vi "002_Control Panel.vi"(11 "Queue Ref In":T1={"UI"=refnum, "Message"=refnum, "Data"=refnum, "Caller"=refnum, "Name"="000 Common", "Data Path"=path "", "Class Path"=path "", "SubPanel"=refnum, "Project Name"="", "MNT"="", "Title"="", "Data Source"=refnum, "Queue List"={}, "VI"=refnum, "UE"=refnum}) -> ()   [LabVIEW 2020]
uses:
  Alin/QMH/000 Module Data Type.ctl
  Alin/QMH/Queue Message.ctl
  <vilib>/Utility/miscctls.llb/LVPointTypeDef.ctl
  0007 Controls/Data Modules.ctl
  0007 Controls/Data Element Single.ctl
  393dfcde-afa0-436b-95a7-8b638b76bd89.vi
  <vilib>/Utility/file.llb/Read Delimited Spreadsheet (string).vi
  <vilib>/Utility/file.llb/Write Delimited Spreadsheet (string).vi
panel:
  in  "Panel Show":bool
  in  "BG3":bool
  in  "BG2":bool
  in  "BG1":bool
  in  "Control Panel":T2
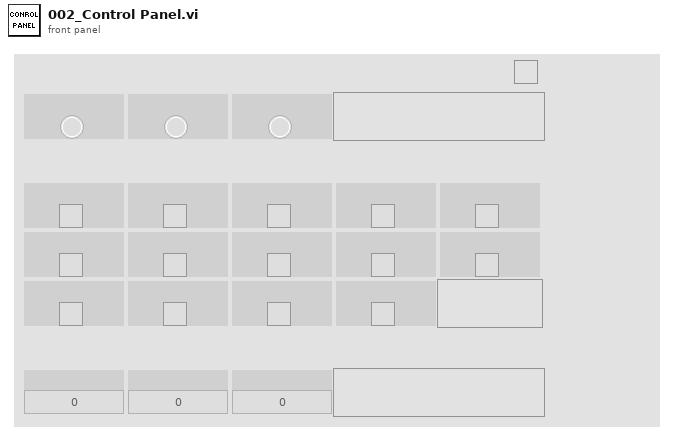
[diagram p1: front panel]
types:
  T1 = typedef "000 Module Data Type.ctl" = cluster{"UI":refnum<queue>, "Message":refnum<queue>, "Data":refnum<queue>, "Caller":refnum<queue>, "Name":string, "Data Path":path, "Class Path":path, "SubPanel":refnum<vi>, "Project Name":string, "MNT":string, "Title":string, "Data Source":refnum<queue>, "Queue List":map{string, refnum<queue>}, "VI":refnum<vi>, "UE":refnum<user-event>}
  T2 = cluster{"System Status":cluster{"Module Name":string, "Data":cluster{"Identifier":string, "Name":string, "Value":bool}[][]}, "Switch":cluster{"Module Name":string, "Data":cluster{"Identifier":string, "Name":string, "Value":bool}[][]}, "Parameter":cluster{"Module Name":string, "Data":cluster{"Identifier":string, "Name":string, "Value":dbl}[][]}}
  T3 = cluster{"Queue":T1, "Array":cluster{string[][]}[], "Active Row":i32, "Delay":cluster{"Count Time(ms)":u32, "Delay Time(ms)":u32, "Next":string}, "Data":cluster{cluster{"Identifier":string, "Name":string, "Value":variant}[][]}[]}
  T4 = typedef "SDQ Data Type.ctl" = cluster{"CAN Length":string, "CAN Name":string, "CAN ID":string, "CAN Type":string, "Test Item":string, "Byte Order":string, "Instruction":string, "Control Type":string, "Group":string, "Offset":dbl, "Coefficient":dbl, "Write Enable":bool, "Lable Type":string, "Key?":string, "Set Value":string, "Upper":dbl, "Lower":dbl, "Unit":string, "Formula":string, "Test Item Type":string, "Length":i32, "Address":string, "Name":string, "Identifier":string, "Data Type":string, "Enumerate?":string, "Enumerate List":string, "Data":string, "Source":string}
  T5 = cluster{cluster{"Identifier":string, "Name":string, "Value":variant}[][]}[]
  T6 = cluster{cluster{"Identifier":string, "Name":string, "Value":variant}[][]}
  T7 = cluster{"Identifier":string, "Name":string, "Value":bool}[][]
  T8 = cluster{"Identifier":string, "Name":string, "Value":dbl}[][]
  T9 = cluster{"Identifier":string, "Name":string, "Value":variant}[][]
  T10 = cluster{"Identifier":string, "Name":string, "Value":bool}
  T11 = cluster{"Identifier":string, "Name":string, "Value":dbl}
  T12 = typedef "eventvkey.ctl" = enum16{"ASCII", "Enter", "Return", "Shift", "Ctrl", "Alt", "Cmd", "Opt", "Caps", "NumLock", "Clear", "Break", "Up", "Down", "Left", "Right", "Insert", "Delete", "Home", "End", "PageUp", "PageDown", "Escape", "Help", "Pause", "ScrollLock", "F1", "F2", "F3", "F4", "F5", "F6", "F7", "F8", "F9", "F10", "F11", "F12", "F13", "F14", "F15", "F16", "F17", "F18", "F19", "F20", "F21", "F22", "F23", "F24", "Play", "VolumeUp", "VolumeDown", "Mute", "Two Byte Char"}
  T13 = cluster{"Shift":bool, "Ctrl":bool, "Alt":bool, "Cmd":bool, "Opt":bool}
  T14 = cluster{"Queue":T1, "Control Panel":refnum<vi>, "Main":refnum<vi>}
  T15 = enum16{"Always On", "Always Off", "Off While Running"}
  T16 = typedef "LVPointTypeDef.ctl" = cluster{"Horizontal":i16, "Vertical":i16}
  T17 = typedef "Data Modules.ctl" = cluster{"Names":cluster{"Module Name":string, "Set Value":string, "Real Value":string, "FB Value":string, "Unit":string, "Identifier":string, "IdentifierW":string, "Decimal":string, "AS":bool, "AR":bool, "Con":bool}, "Data":T18[], "Digit":dbl}
  T18 = typedef "Data Element Single.ctl" = cluster{"Name":string, "Set Value":string, "Real Value":string, "FB Value":string, "Unit":string, "Identifier":string, "Write Name":string, "Decimal":u16, "AS":bool, "AR":bool, "ALM":bool, "Up":bool, "Down":bool}
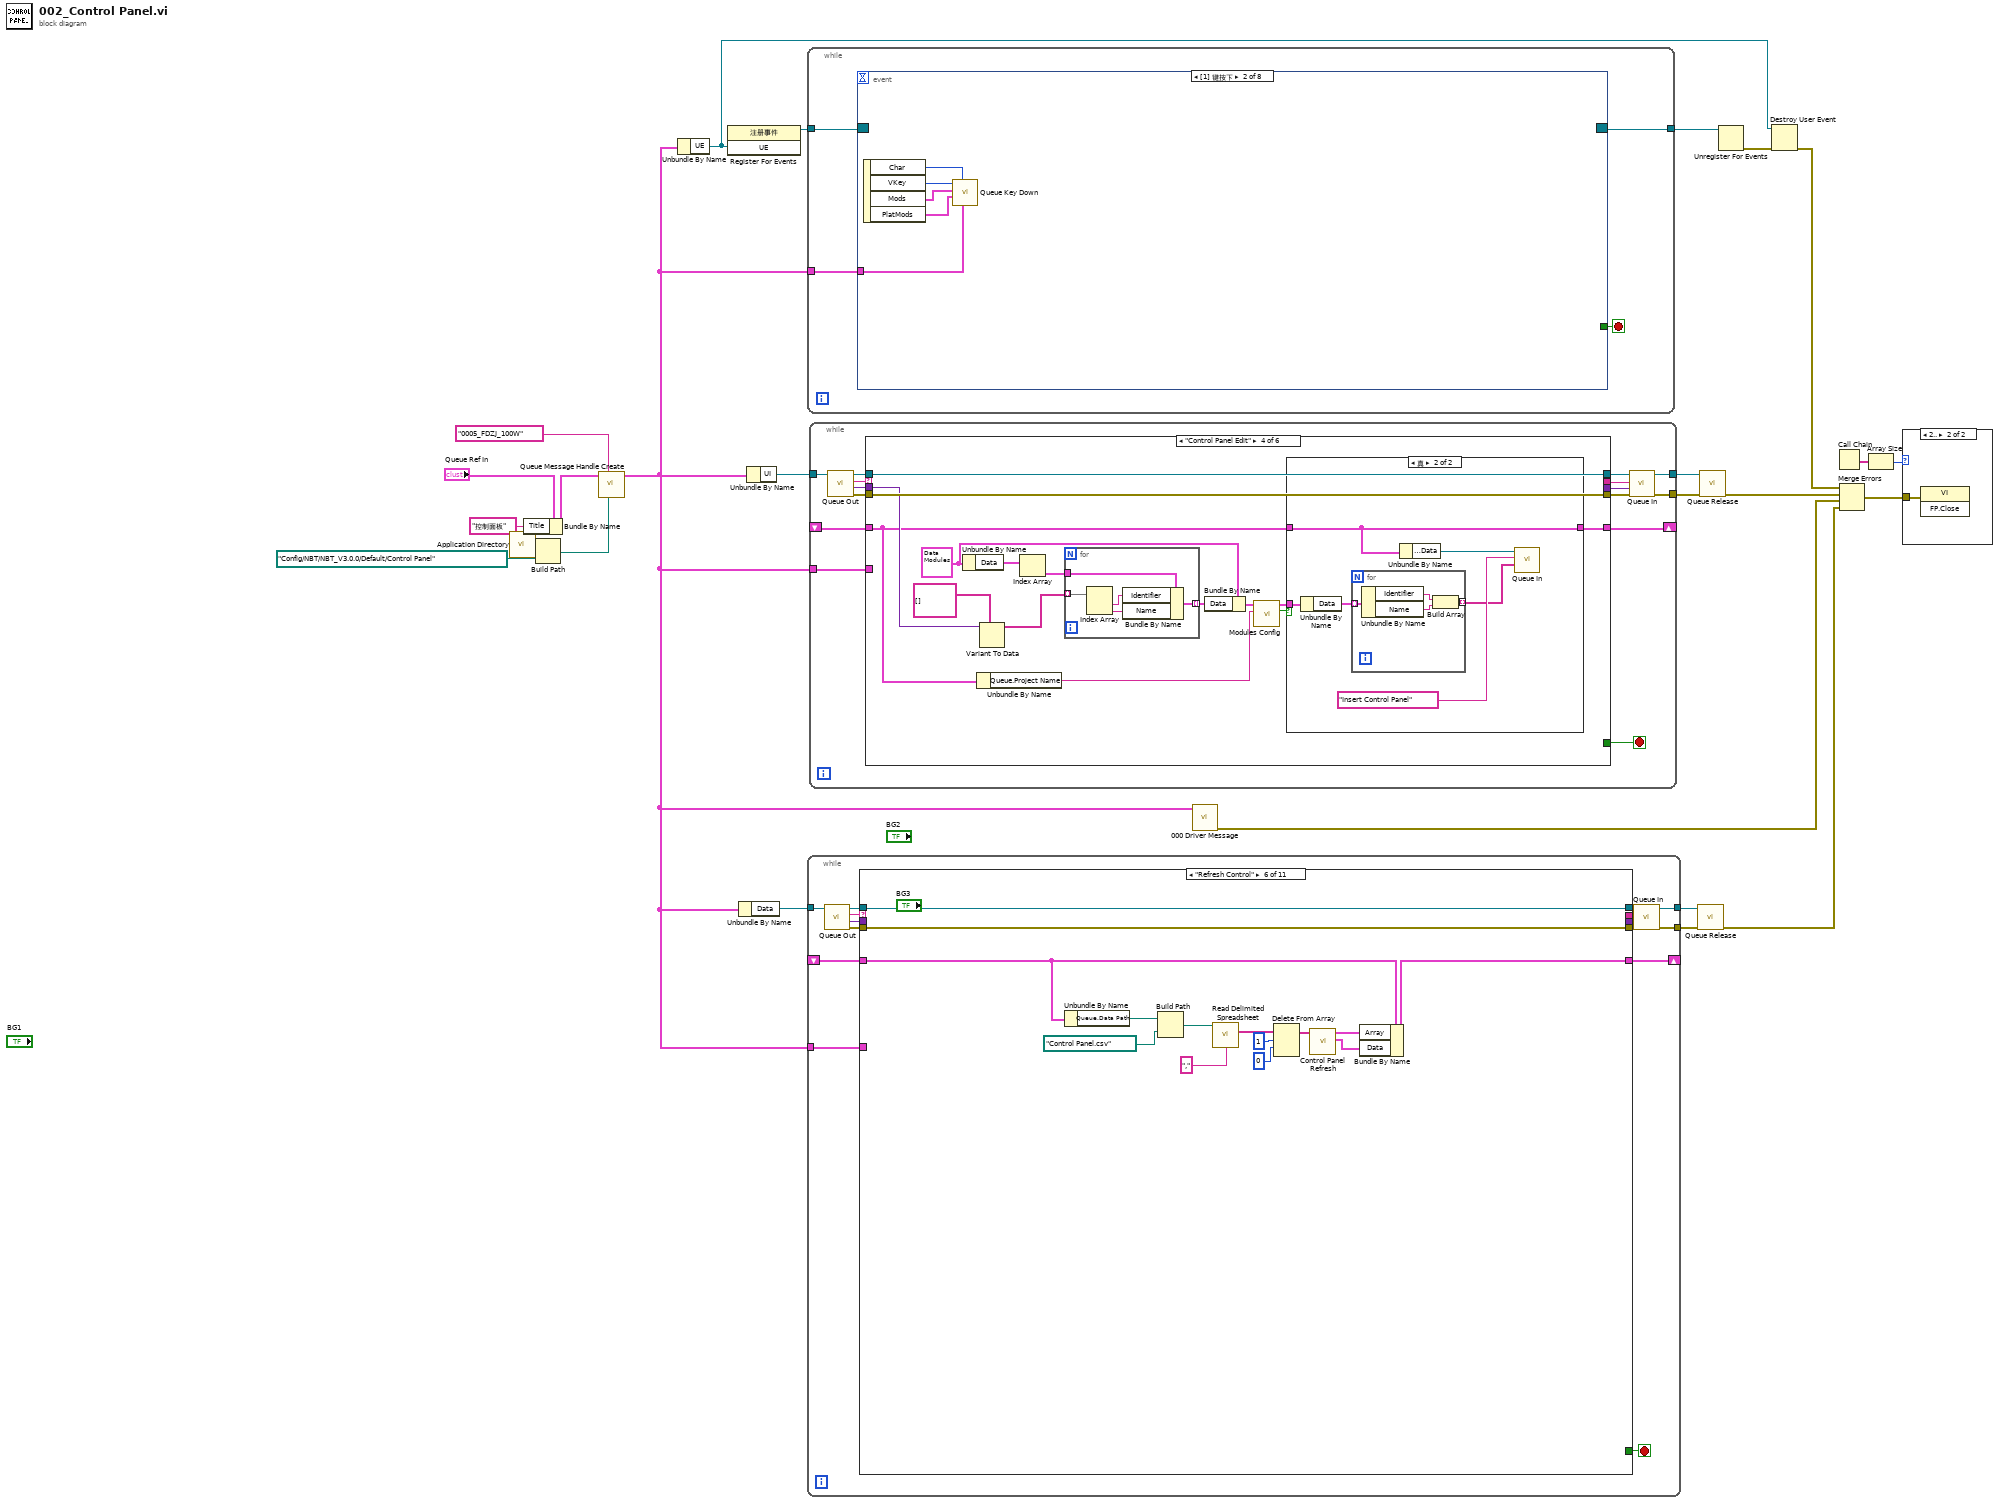
[diagram p0: block diagram]
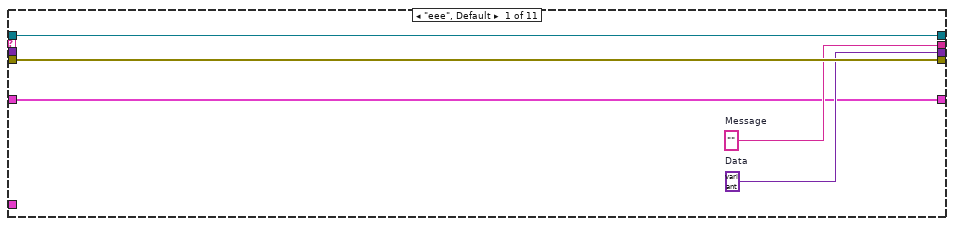
[diagram p2: hidden frame]
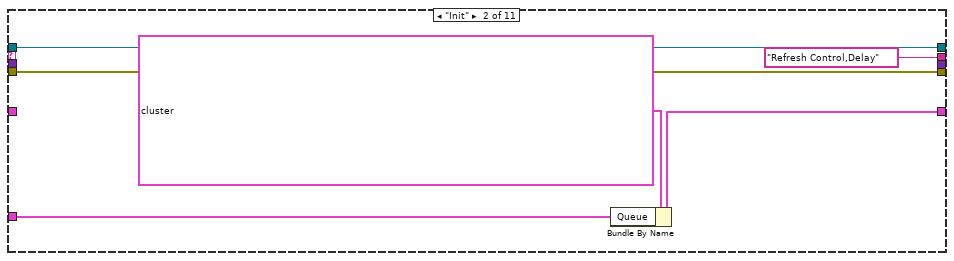
[diagram p3: hidden frame]
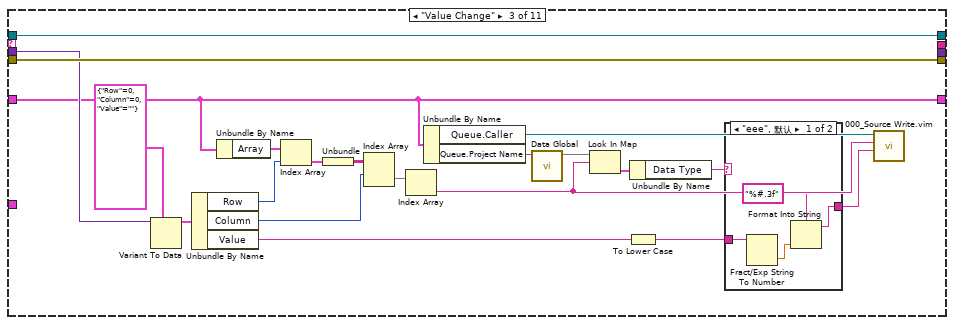
[diagram p4: hidden frame]
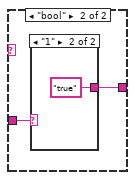
[diagram p5: hidden frame]
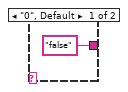
[diagram p6: hidden frame]
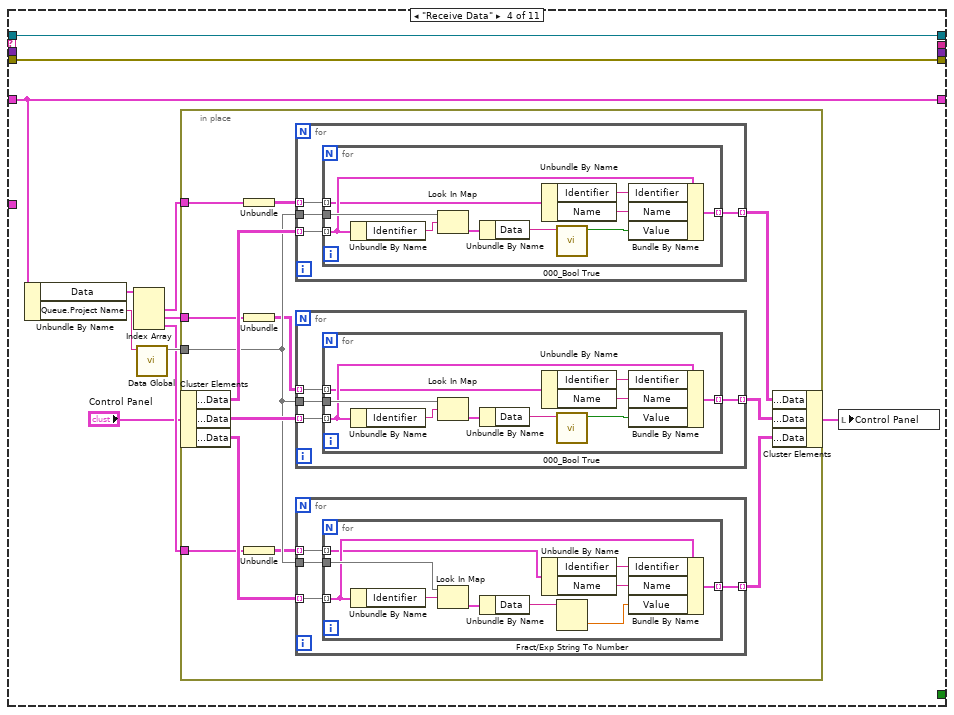
[diagram p7: hidden frame]
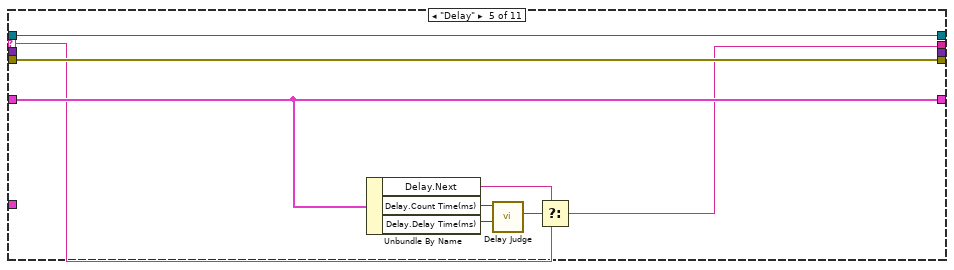
[diagram p8: hidden frame]
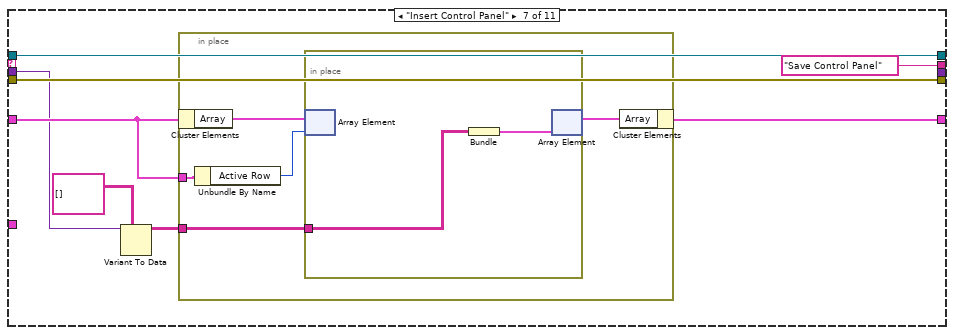
[diagram p9: hidden frame]
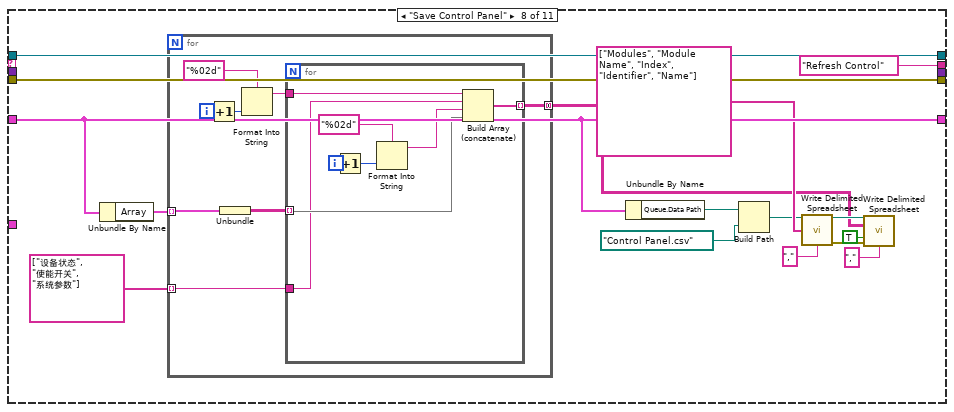
[diagram p10: hidden frame]
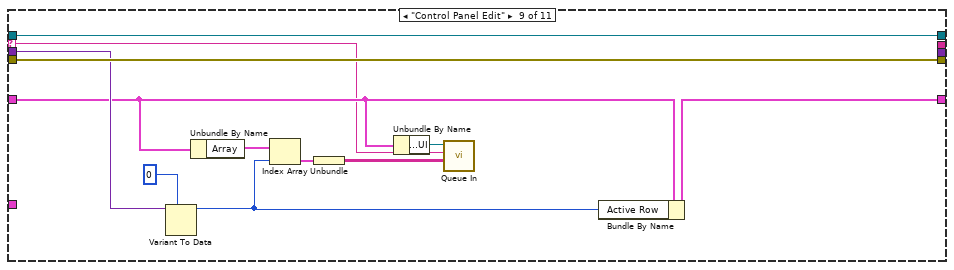
[diagram p11: hidden frame]
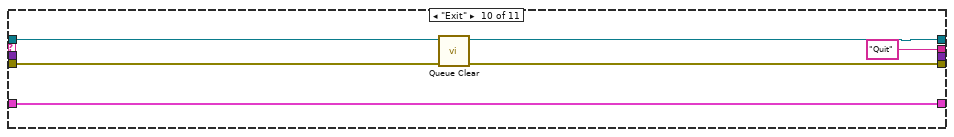
[diagram p12: hidden frame]
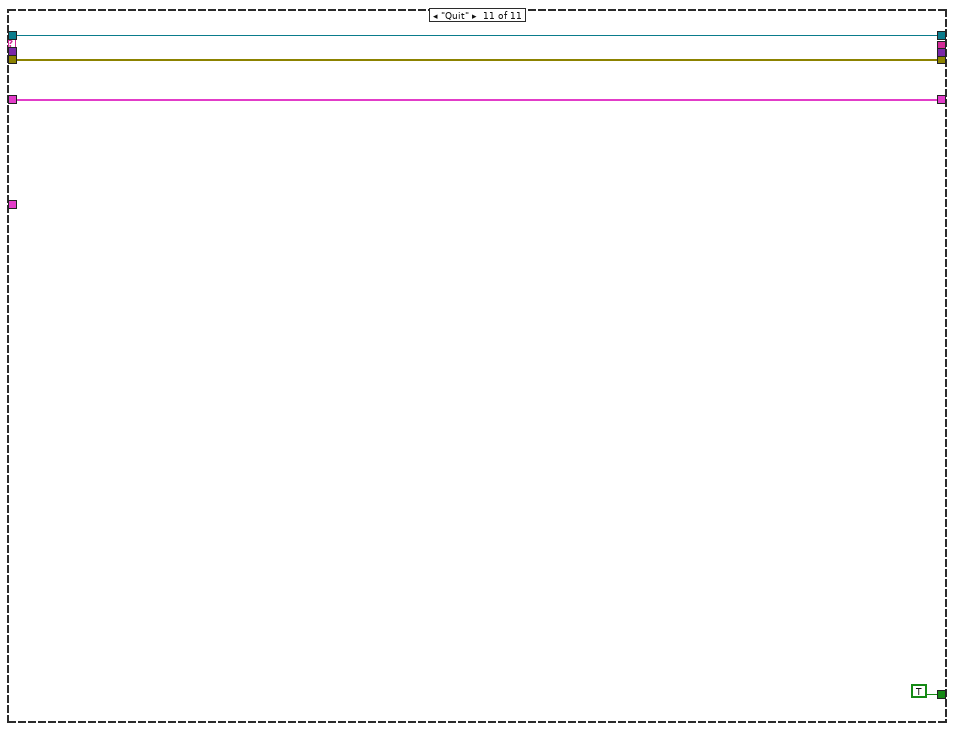
[diagram p13: hidden frame]
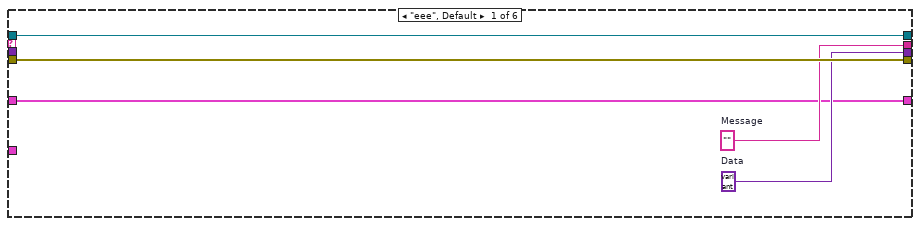
[diagram p15: hidden frame]
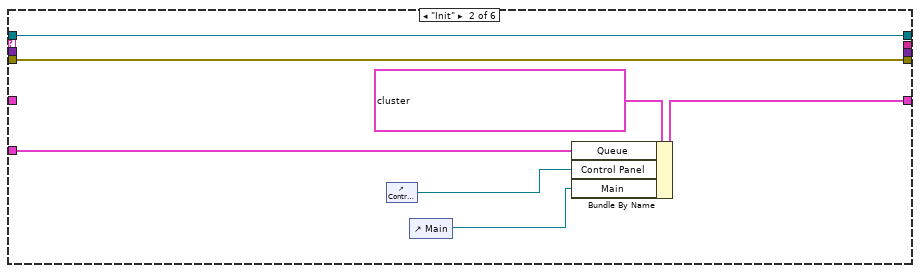
[diagram p16: hidden frame]
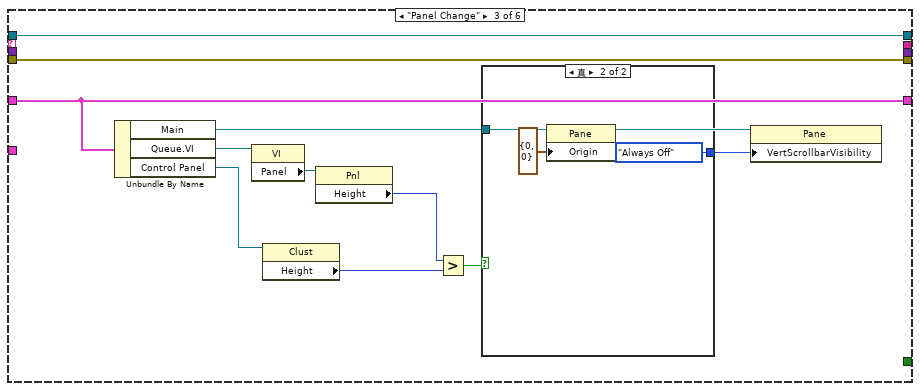
[diagram p17: hidden frame]
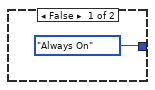
[diagram p18: hidden frame]
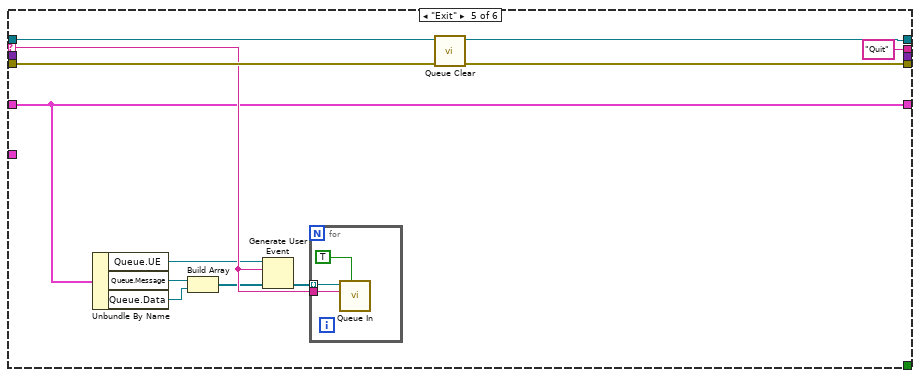
[diagram p20: hidden frame]
diagram:
  n1 = call <vilib>:"Application Directory.vi"() -> ("Application Directory"=w3:path)
  n2 = Bundle By Name(cluster="Queue Ref In", "Title"="控制面板") -> (w8:T1)
  n3 = Build Path(base path=w3, name or relative path=path "Config/NBT/NBT_V3.0.0/Default/Control Panel" ("路径")) -> (appended path=w1:path)
  n4 = call "Queue Message Handle Create.vi"("Data Path"=w1, "Project Name"="0005_FDZJ_100W", "Queue Ref In"=w8) -> ("Queue Ref Out"=w5:T1)  [unwired: 7 in, 1 out]
  n5 = Unbundle By Name(w5) -> ("UE"=w6:refnum<user-event>)
  n6 = register-events(w6) -> (reference out=w9:refnum<event-registration>)  [unwired: 2 in, 1 out]
  n7 = Unbundle By Name(w5) -> ("Data"=w22:refnum<queue>)
  n8 = Unbundle By Name(w5) -> ("UI"=w14:refnum<queue>)
  n9 = while {
    tunnel: w22 -> [w36]
    tunnel: [w33] -> w20
    tunnel: [w32] -> w21
    tunnel: w5 -> [w28]
    shift-right: [w27] -> _
    shift-left: _ -> [w26]
    stop <- w40 stop-if-true
    n10 = call "Queue Out.vi"("Queue In"=w36) -> ("error out"=w39:errorcluster, "Data"=w37:variant, "Message"=w38:string, "Queue Out"=w35:refnum<queue>)  [unwired: 6 in, 1 out]
    n11 = case shown="\"Refresh Control\"" w38 {
      selector: w38 -> [_ _ _ _ w148 _ _ _ w219 _ _]
      tunnel: w35 -> [w45 w51 w72 w91 w155 w169 w177 w200 w228 w233 w237]
      tunnel: w39 -> [w44 w50 w71 w90 w154 w168 w176 w199 w227 w231 w238]
      tunnel: [w45 w51 w72 w91 w155 w169 w177 w200 w228 w232 w237] -> w34
      tunnel: [w44 w50 w71 w90 w154 w168 w176 w199 w227 w230 w238] -> w31
      tunnel: [w43 "Refresh Control,Delay" ("Message") _ _ w147 _ "Save Control Panel" ("Message") "Refresh Control" ("Message") _ "Quit" _] -> w30
      tunnel: [_ _ _ _ _ _ _ _ _ _ TRUE] -> w40
      tunnel: [w42 _ _ _ _ _ _ _ _ _ _] -> w29
      tunnel: w37 -> [_ _ w70 _ _ _ w172 _ w226 _ _]
      tunnel: w28 -> [_ w47 _ _ _ _ _ _ _ _ _]
      tunnel: [w41 w46 w61 w89 w149 w166 w174 w195 w218 w229 w235] -> w27
      tunnel: w26 -> [w41 _ w61 w89 w149 w164 w173 w195 w222 w229 w235]
      frame "eee", Default {
        w42 = variant  # Data
        w43 = ""  # Message
      }
      frame "Init" {
        n12 = Bundle By Name(cluster=T3 {"Queue"={"UI"=refnum, "Message"=refnum, "Data"=refnum, "Caller"=refnum, "Name"="000 Common", "Data Path"=path "", "Class Path"=path "", "SubPanel"=refnum, "Project Name"="", "MNT"="", "Title"="", "Data Source"=refnum, "Queue List"={}, "VI"=refnum, "UE"=refnum}, "Array"=[], "Active Row"=0, "Delay"={"Count Time(ms)"=500, "Delay Time(ms)"=250, "Next"="Receive Data,Delay"}, "Data"=[]}, "Queue"=w47) -> (w46:T3)
      }
      frame "Value Change" {
        n13 = Variant To Data(type=cluster{"Row":i32, "Column":i32, "Value":string} {"Row"=0, "Column"=0, "Value"=""} ("簇"), Variant=w70) -> (data=w68:cluster{"Row":i32, "Column":i32, "Value":string})  [unwired: 1 in, 1 out]
        n14 = Unbundle By Name(w68) -> ("Row"=w64:i32, "Column"=w63:i32, "Value"=w56:string)
        n15 = Unbundle By Name(w61) -> ("Array"=w67:cluster{string[][]}[])
        n16 = Index Array(array=w67, index=w64) -> (element=w66:cluster{string[][]})
        n17 = Unbundle(w66) -> (w65:string[][])
        n18 = Index Array(array=w65, index (row)=w63) -> (element=w62:string[])  [unwired: 1 in]
        n19 = Index Array(array=w62) -> (element=w53:string)  [unwired: 1 in]
        n20 = Unbundle By Name(w61) -> ("Queue.Caller"=w54:refnum<queue>, "Queue.Project Name"=w60:string)
        n21 = call "Data Global.vi"("Name"=w60) -> ("Data Out"=w59:map{string, T4})  [unwired: 7 in, 3 out]
        n22 = Look In Map(map=w59, key=w53) -> (value=w58:T4)  [unwired: 1 in, 1 out]
        n23 = To Lower Case(string=w56) -> (all lower case string=w55:string)
        n24 = Unbundle By Name(w58) -> ("Data Type"=w57:string)
        n25 = case shown="\"eee\", 默认" w57 {
          tunnel: w55 -> [w76 w78]
          tunnel: [w73 w77] -> w52
          frame "eee", Default {
            n26 = Fract/Exp String To Number(string=w76) -> (number=w74:dbl)  [unwired: 3 in, 1 out]
            n27 = Format Into String(format string="%#.3f" ("格式字符串"), w74) -> (resulting string=w73:string)  [unwired: 2 in, 1 out]
          }
          frame "bool" {
            n28 = case shown="\"1\"" w78 {
              tunnel: ["false" "true"] -> w77
              frame "0", Default {
              }
              frame "1" {
              }
            }
          }
        }
        n29 = call "000_Source Write.vim"("Data"=w52, "Name"=w53, "Queue In"=w54) -> ()  [unwired: 6 in, 3 out]
      }
      frame "Receive Data" {
        n30 = Unbundle By Name(w89) -> ("Data"=w82:T5, "Queue.Project Name"=w81:string)
        n31 = Index Array(array=w82) -> (element #1=w87:T6, element #2=w86:T6, element #3=w85:T6)  [unwired: 3 in]
        n32 = call "Data Global.vi"("Name"=w81) -> ("Data Out"=w88:map{string, T4})  [unwired: 7 in, 3 out]
        n33 = in-place {
          in-place-border: w88 -> [w99]
          in-place-border: w87 -> [w97]
          in-place-border: w86 -> [w96]
          in-place-border: w85 -> [w95]
          n34 = in-place-cluster #1("Control Panel") -> ("System Status.Data"=w104:T7, "Switch.Data"=w102:T7, "Parameter.Data"=w100:T8)
          n35 = Unbundle(w97) -> (w94:T9)
          n36 = Unbundle(w96) -> (w93:T9)
          n37 = Unbundle(w95) -> (w92:T9)
          n38 = for {
            tunnel: w104 -> [w136] mode=indexing
            tunnel: w99 -> [w135]
            tunnel: [w134] -> w103 mode=indexing
            tunnel: w94 -> [w133] mode=indexing
            n39 = for {
              tunnel: w136 -> [w141] mode=indexing
              tunnel: w135 -> [w146]
              tunnel: [w140] -> w134 mode=indexing
              tunnel: w133 -> [w139] mode=indexing
              n40 = Unbundle By Name(w141) -> ("Identifier"=w145:string)
              n41 = Look In Map(map=w146, key=w145) -> (value=w144:T4)  [unwired: 1 in, 1 out]
              n42 = Unbundle By Name(w144) -> ("Data"=w143:string)
              n43 = Unbundle By Name(w139) -> ("Identifier"=w138:string, "Name"=w137:string)
              n44 = call "000_Bool True.vi"("Bool String"=w143) -> ("True"=w142:bool)  [unwired: 8 in, 2 out]
              n45 = Bundle By Name(cluster=w141, "Identifier"=w138, "Name"=w137, "Value"=w142) -> (w140:T10)
            }
          }
          n46 = for {
            tunnel: w102 -> [w122] mode=indexing
            tunnel: w99 -> [w121]
            tunnel: [w120] -> w101 mode=indexing
            tunnel: w93 -> [w119] mode=indexing
            n47 = for {
              tunnel: w122 -> [w127] mode=indexing
              tunnel: w121 -> [w132]
              tunnel: [w126] -> w120 mode=indexing
              tunnel: w119 -> [w125] mode=indexing
              n48 = Unbundle By Name(w127) -> ("Identifier"=w131:string)
              n49 = Look In Map(map=w132, key=w131) -> (value=w130:T4)  [unwired: 1 in, 1 out]
              n50 = Unbundle By Name(w130) -> ("Data"=w129:string)
              n51 = Unbundle By Name(w125) -> ("Identifier"=w124:string, "Name"=w123:string)
              n52 = call "000_Bool True.vi"("Bool String"=w129) -> ("True"=w128:bool)  [unwired: 8 in, 2 out]
              n53 = Bundle By Name(cluster=w127, "Identifier"=w124, "Name"=w123, "Value"=w128) -> (w126:T10)
            }
          }
          n54 = for {
            tunnel: w100 -> [w108] mode=indexing
            tunnel: w99 -> [w107]
            tunnel: [w106] -> w98 mode=indexing
            tunnel: w92 -> [w105] mode=indexing
            n55 = for {
              tunnel: w108 -> [w115] mode=indexing
              tunnel: w107 -> [w118]
              tunnel: [w114] -> w106 mode=indexing
              tunnel: w105 -> [w111] mode=indexing
              n56 = Unbundle By Name(w115) -> ("Identifier"=w117:string)
              n57 = Look In Map(map=w118, key=w117) -> (value=w116:T4)  [unwired: 1 in, 1 out]
              n58 = Unbundle By Name(w116) -> ("Data"=w113:string)
              n59 = Unbundle By Name(w111) -> ("Identifier"=w110:string, "Name"=w109:string)
              n60 = Fract/Exp String To Number(string=w113) -> (number=w112:dbl)  [unwired: 3 in, 1 out]
              n61 = Bundle By Name(cluster=w115, "Identifier"=w110, "Name"=w109, "Value"=w112) -> (w114:T11)
            }
          }
          n62 = in-place-cluster #1("System Status.Data"=w103, "Switch.Data"=w101, "Parameter.Data"=w98) -> (w84:T2)
        }
        n63 = local write "Control Panel"(w84) -> ()
      }
      frame "Delay" {
        n64 = Unbundle By Name(w149) -> ("Delay.Next"=w153:string, "Delay.Count Time(ms)"=w150:u32, "Delay.Delay Time(ms)"=w151:u32)
        n65 = call "Delay Judge.vi"("Delay Time(ms)"=w151, "Count Time(ms)"=w150) -> ("Time Out?"=w152:bool)  [unwired: 5 in, 4 out]
        n66 = Select(t=w153, s=w152, f=w148) -> (s? t:f=w147:string)
      }
      frame "Refresh Control" {
        n67 = Unbundle By Name(w164) -> ("Queue.Data Path"=w163:path)
        n68 = Build Path(base path=w163, name or relative path=path "Control Panel.csv" ("file path (dialog if empty)")) -> (appended path=w161:path)
        n69 = call-poly <vilib>:"Read Delimited Spreadsheet.vi"("file path (dialog if empty)"=w161, "delimiter (\\t)"="," ("delimiter (\\t)")) -> ("all rows"=w158:string[][])  [unwired: 8 in, 5 out]
        n70 = Delete From Array(array=w158, length=1 ("长度"), index (row)=0 ("索引 (行)")) -> (array with subset deleted=w157:string[][])  [unwired: 1 in, 1 out]
        n71 = call "Control Panel Refresh.vi"("Data In"=w157) -> ("Data"=w156:T5, "Array"=w167:cluster{string[][]}[])  [unwired: 9 in]
        n72 = Bundle By Name(cluster=w164, "Array"=w167, "Data"=w156) -> (w166:T3)
      }
      frame "Insert Control Panel" {
        n73 = Variant To Data(type=string[][] [], Variant=w172) -> (data=w170:string[][])  [unwired: 1 in, 1 out]
        n74 = in-place {
          in-place-border: w173 -> [w181]
          in-place-border: w170 -> [w178]
          n75 = in-place-cluster #2(w173) -> ("Array"=w182:cluster{string[][]}[])
          n76 = Unbundle By Name(w181) -> ("Active Row"=w180:i32)
          n77 = in-place {
            in-place-border: w178 -> [w184]
            n78 = in-place-array #3(w182, w180) -> ()  [unwired: 1 out]
            n79 = Bundle(w184) -> (w183:cluster{string[][]})  [unwired: 1 in]
            n80 = in-place-array #3(w183) -> (w179:cluster{string[][]}[])  [unwired: 1 out]
          }
          n81 = in-place-cluster #2("Array"=w179) -> (w174:T3)
        }
      }
      frame "Save Control Panel" {
        n82 = Unbundle By Name(w195) -> ("Array"=w198:cluster{string[][]}[])
        n83 = for {
          tunnel: w198 -> [w208] mode=indexing
          tunnel: [w203] -> w186 mode=concatenating
          tunnel: string[] ["设备状态", "使能开关", "系统参数"] -> [w202] mode=indexing
          i -> [w205]
          n84 = Increment(x=w205) -> (x+1=w201:i32)
          n85 = Unbundle(w208) -> (w207:string[][])
          n86 = Format Into String(format string="%02d" ("格式字符串"), w201) -> (resulting string=w204:string)  [unwired: 2 in, 1 out]
          n87 = for {
            tunnel: w207 -> [w213] mode=indexing
            tunnel: w204 -> [w211]
            tunnel: [w212] -> w203 mode=indexing
            tunnel: w202 -> [w210]
            i -> [w215]
            n88 = Increment(x=w215) -> (x+1=w209:i32)
            n89 = Format Into String(format string="%02d" ("格式字符串"), w209) -> (resulting string=w214:string)  [unwired: 2 in, 1 out]
            n90 = Build Array (concatenate)(w211, w210, w214, w213) -> (w212:string[])
          }
        }
        n91 = Unbundle By Name(w195) -> ("Queue.Data Path"=w197:path)
        n92 = Build Path(base path=w197, name or relative path=path "Control Panel.csv" ("file path (dialog if empty)")) -> (appended path=w187:path)
        n93 = call-poly <vilib>:"Write Delimited Spreadsheet.vi"("file path (dialog if empty)"=w187, "1D data"=string[] ["Modules", "Module Name", "Index", "Identifier", "Name"], "delimiter (\\t)"="," ("delimiter (\\t)")) -> ("new file path (Not A Path if cancelled)"=w191:path, "error out"=w190:errorcluster)  [unwired: 11 in]
        n94 = call-poly <vilib>:"Write Delimited Spreadsheet.vi"("file path (dialog if empty)"=w191, "2D data"=w186, "append to file? (new file:F)"=TRUE, "error in (no error)"=w190, "delimiter (\\t)"="," ("delimiter (\\t)")) -> ()  [unwired: 9 in, 2 out]
      }
      frame "Control Panel Edit" {
        n95 = Variant To Data(type=0 ("元素索引"), Variant=w226) -> (data=w217:i32)  [unwired: 1 in, 1 out]
        n96 = Unbundle By Name(w222) -> ("Array"=w224:cluster{string[][]}[])
        n97 = Index Array(array=w224, index=w217) -> (element=w223:cluster{string[][]})
        n98 = Unbundle(w223) -> (w220:string[][])
        n99 = Unbundle By Name(w222) -> ("Queue.UI"=w221:refnum<queue>)
        n100 = call "Queue In.vi"("Data"=w220, "Message"=w219, "Queue In"=w221) -> ()  [unwired: 7 in, 2 out]
        n101 = Bundle By Name(cluster=w222, "Active Row"=w217) -> (w218:T3)
      }
      frame "Exit" {
        n102 = call "Queue Clear.vi"("error in (no error)"=w231, "Queue In"=w233) -> ("error out"=w230:errorcluster, "Queue Out"=w232:refnum<queue>)  [unwired: 8 in]
      }
      frame "Quit" {
      }
    }
    n103 = call "Queue In.vi"("error in (no error)"=w31, "Data"=w29, "Message"=w30, "Queue In"=w34) -> ("error out"=w32:errorcluster, "Queue Out"=w33:refnum<queue>)  [unwired: 6 in]
  }
  n104 = while {
    tunnel: w9 -> [w242]
    tunnel: [w240] -> w10
    tunnel: w5 -> [w239]
    stop <- w241 stop-if-true
    n105 = event shown="[1] 键按下" {
      selector: w242 -> [_ _ _ _ _ _ _ _]
      dyn-events: [_ _ _ _ _ _ _ _] -> w240
      timeout: _ -> [_ _ _ _ _ _ _ _]
      tunnel: [_ _ _ _ _ w278 _ _] -> w241
      tunnel: w239 -> [_ w246 w250 w253 w268 _ w284 w296]
      event Timeout {
        n106 = event-data() -> ()  [unwired: 1 in, 1 out]
      }
      event Key Down {
        n107 = event-data() -> ("Char"=w247:i16, "VKey"=w245:T12, "Mods"=w244:cluster{"Num Pad":bool, "Menu Key":bool}, "PlatMods"=w243:T13)  [unwired: 1 in]
        n108 = call "Queue Key Down.vi"("Queue Ref Out"=w246, "C"=w247, "Platform Key"=w243, "Group Key"=w244, "V Key"=w245) -> ()  [unwired: 6 in, 1 out]
      }
      event Panel Resize {
        n109 = event-data() -> ()  [unwired: 1 in, 1 out]
        n110 = Unbundle By Name(w250) -> ("UI"=w249:refnum<queue>)
        n111 = call "Queue In.vi"("Message"="Panel Change", "Queue In"=w249) -> ()  [unwired: 8 in, 2 out]
      }
      event "Control Panel.System Status", "Control Panel.Switch", "Control Panel.Parameter": Mouse Down {
        n112 = event-data() -> ("CtlRef"=w252:refnum<vi>, "Mods.Double Click"=w251:bool)  [unwired: 1 in]
        n113 = case shown="真" w251 {
          tunnel: w253 -> [_ w261]
          tunnel: w252 -> [_ w258]
          frame False {
          }
          frame True {
            n114 = Unbundle By Name(w261) -> ("Data"=w260:refnum<queue>)
            n115 = property class="Clust"(reference=w258) -> ("Label.Text"=w256:string)  [unwired: 1 in, 2 out]
            n116 = Search 1D Array(1D array=string[] ["System Status", "Switch", "Parameter"], element=w256) -> (index of element=w255:i32)  [unwired: 1 in]
            n117 = call "Queue In.vi"("First"=TRUE, "Data"=w255, "Message"="Control Panel Edit", "Queue In"=w260) -> ()  [unwired: 6 in, 2 out]
          }
        }
      }
      event "Control Panel.System Status", "Control Panel.Switch", "Control Panel.Parameter": Value Change {
        n118 = event-data() -> ("CtlRef"=w273:refnum<vi>, "OldVal"=w277:variant, "NewVal"=w276:variant)  [unwired: 1 in]
        n119 = call "Cluster Get Control Value Change.vi"("variant 2"=w276, "variant 1"=w277) -> ("Value"=w262:string, "Index"=w272:i32)  [unwired: 6 in, 2 out]
        n120 = property class="Clust"(reference=w273) -> ("Label.Text"=w274:string)  [unwired: 1 in, 2 out]
        n121 = Quotient & Remainder(x=w272, y=3) -> (floor(x/y)=w269:i32)  [unwired: 1 out]
        n122 = Search 1D Array(1D array=string[] ["System Status", "Switch", "Parameter"], element=w274) -> (index of element=w270:i32)  [unwired: 1 in]
        n123 = Decrement(x=w269) -> (x-1=w263:i32)
        n124 = Unbundle By Name(w268) -> ("Data"=w267:refnum<queue>)
        n125 = Bundle(cluster=cluster{"Row":i32, "Column":i32, "Value":string} {"Row"=0, "Column"=0, "Value"=""} ("簇"), "Row"=w270, "Column"=w263, "Value"=w262) -> (w265:cluster{"Row":i32, "Column":i32, "Value":string})
        n126 = call "Queue In.vi"("Data"=w265, "Message"="Value Change", "Queue In"=w267) -> ()  [unwired: 7 in, 2 out]
      }
      event User Event {
        n127 = event-data() -> ("Message"=w280:string)  [unwired: 1 in]
        n128 = Equal?(x=w280, y="Exit") -> (x = y?=w278:bool)
      }
      event Panel Close? {
        n129 = event-data() -> ()  [unwired: 1 in, 1 out]
        n130 = Call Chain() -> (call chain=w286:string[])
        n131 = Array Size(array=w286) -> (size(s)=w285:i32)
        n132 = case shown="1" w285 {
          tunnel: w284 -> [w290 w293]
          tunnel: [w289 w292] -> w283
          tunnel: ["Panel Hidden" ("Message") "Exit Prepare" ("Message")] -> w282
          frame 2, Default {
            n133 = Unbundle By Name(w290) -> ("Message"=w289:refnum<queue>)
          }
          frame 1 {
            n134 = Unbundle By Name(w293) -> ("Message"=w292:refnum<queue>)
          }
        }
        n135 = call "Queue In.vi"("First"=TRUE, "Message"=w282, "Queue In"=w283) -> ()  [unwired: 7 in, 2 out]
        n136 = event-data("Discard?"=TRUE ("放弃？")) -> ()  [unwired: 1 in, 1 out]
      }
      event "Panel Show": Value Change {
        n137 = event-data() -> ("CtlRef"=w297:refnum<vi>)  [unwired: 1 in]
        n138 = Unbundle By Name(w296) -> ("Message"=w295:refnum<queue>)
        n139 = property class="Bool"(reference=w297) -> ("Label.Text"=w294:string)  [unwired: 1 in, 2 out]
        n140 = call "Queue In.vi"("Message"=w294, "Queue In"=w295) -> ()  [unwired: 8 in, 2 out]
      }
    }
  }
  n141 = while {
    tunnel: w14 -> [w308]
    tunnel: [w305] -> w12
    tunnel: [w304] -> w13
    tunnel: w5 -> [w300]
    shift-right: [w299] -> _
    shift-left: _ -> [w298]
    stop <- w312 stop-if-true
    n142 = call "Queue Out.vi"("Queue In"=w308) -> ("error out"=w311:errorcluster, "Data"=w309:variant, "Message"=w310:string, "Queue Out"=w307:refnum<queue>)  [unwired: 6 in, 1 out]
    n143 = case shown="\"Control Panel Edit\"" w310 {
      selector: w310 -> [_ _ _ _ w376 _]
      tunnel: w307 -> [w317 w324 w335 w354 w380 w387]
      tunnel: w311 -> [w316 w323 w334 w353 w378 w388]
      tunnel: [w317 w324 w335 w354 w379 w387] -> w306
      tunnel: [w316 w323 w334 w353 w377 w388] -> w303
      tunnel: [w315 _ _ _ "Quit" _] -> w302
      tunnel: [_ _ _ _ _ TRUE] -> w312
      tunnel: [w314 _ _ _ _ _] -> w301
      tunnel: w309 -> [_ _ _ w352 _ _]
      tunnel: w300 -> [_ w320 _ _ _ _]
      tunnel: [w313 w321 w333 w350 w375 w385] -> w299
      tunnel: w298 -> [w313 _ w333 w341 w375 w385]
      frame "eee", Default {
        w314 = variant  # Data
        w315 = ""  # Message
      }
      frame "Init" {
        n144 = control-ref of="Control Panel"() -> (w319:refnum<vi>)
        n145 = control-ref of="Main"() -> (w318:refnum<vi>)
        n146 = Bundle By Name(cluster=T14 {"Queue"={"UI"=refnum, "Message"=refnum, "Data"=refnum, "Caller"=refnum, "Name"="000 Common", "Data Path"=path "", "Class Path"=path "", "SubPanel"=refnum, "Project Name"="", "MNT"="", "Title"="", "Data Source"=refnum, "Queue List"={}, "VI"=refnum, "UE"=refnum}, "Control Panel"=refnum, "Main"=refnum}, "Queue"=w320, "Control Panel"=w319, "Main"=w318) -> (w321:T14)
      }
      frame "Panel Change" {
        n147 = Unbundle By Name(w333) -> ("Main"=w325:refnum<vi>, "Queue.VI"=w331:refnum<vi>, "Control Panel"=w332:refnum<vi>)
        n148 = property class="VI"(reference=w331) -> ("Panel"=w330:refnum<vi>)  [unwired: 1 in, 2 out]
        n149 = property class="Clust"(reference=w332) -> ("Height"=w329:u32)  [unwired: 1 in, 2 out]
        n150 = property class="Pnl"(reference=w330) -> ("Height"=w328:u32)  [unwired: 1 in, 2 out]
        n151 = Greater?(x=w328, y=w329) -> (0:w327:bool)
        n152 = case shown="真" w327 {
          tunnel: [T15."Always On" ("f") T15."Always Off" ("垂直滚动条可见")] -> w326
          tunnel: w325 -> [_ w338]
          frame False {
          }
          frame True {
            n153 = property class="Pane"(reference=w338, "Origin"=T16 {"Horizontal"=0, "Vertical"=0} ("原点")) -> ()  [unwired: 1 in, 2 out]
          }
        }
        n154 = property class="Pane"(reference=w325, "VertScrollbarVisibility"=w326) -> ()  [unwired: 1 in, 2 out]
      }
      frame "Control Panel Edit" {
        w345 = T17 {"Names"={"Module Name"="模块名称", "Set Value"="设置值", "Real Value"="实时值", "FB Value"="反馈值", "Unit"="单位", "Identifier"="标识符", "IdentifierW"="写入标识符", "Decimal"="位数", "AS"=FALSE, "AR"=FALSE, "Con"=FALSE}, "Data"=[], "Digit"=0.0} ("Module01")
        n155 = Unbundle By Name(w345) -> ("Data"=w346:T18[])
        n156 = Unbundle By Name(w341) -> ("Queue.Project Name"=w340:string)
        n157 = Variant To Data(type=string[][] [] ("Data In"), Variant=w352) -> (data=w344:string[][])  [unwired: 1 in, 1 out]
        n158 = Index Array(array=w346) -> (element=w347:T18)  [unwired: 1 in]
        n159 = for {
          tunnel: w344 -> [w359] mode=indexing
          tunnel: w347 -> [w358]
          tunnel: [w355] -> w348 mode=indexing
          n160 = Index Array(array=w359) -> (element #1=w357:string, element #2=w356:string)  [unwired: 2 in]
          n161 = Bundle By Name(cluster=w358, "Identifier"=w357, "Name"=w356) -> (w355:T18)
        }
        n162 = Bundle By Name(cluster=w345, "Data"=w348) -> (w349:T17)
        n163 = call "Modules Config.vi"("Name"=w340, "Module In"=w349) -> ("OK？"=w343:bool, "Module Out"=w342:T17)  [unwired: 8 in]
        n164 = case shown="真" w343 {
          tunnel: w341 -> [w360 w366]
          tunnel: [w360 w366] -> w350
          tunnel: w342 -> [_ w363]
          frame False {
          }
          frame True {
            n165 = Unbundle By Name(w363) -> ("Data"=w362:T18[])
            n166 = for {
              tunnel: w362 -> [w370] mode=indexing
              tunnel: [w367] -> w361 mode=indexing
              n167 = Unbundle By Name(w370) -> ("Identifier"=w369:string, "Name"=w368:string)
              n168 = Build Array(w369, w368) -> (w367:string[])
            }
            n169 = Unbundle By Name(w366) -> ("Queue.Data"=w365:refnum<queue>)
            n170 = call "Queue In.vi"("Data"=w361, "Message"="Insert Control Panel", "Queue In"=w365) -> ()  [unwired: 7 in, 2 out]
          }
        }
      }
      frame "Exit" {
        n171 = Unbundle By Name(w375) -> ("Queue.UE"=w374:refnum<user-event>, "Queue.Message"=w373:refnum<queue>, "Queue.Data"=w372:refnum<queue>)
        n172 = Build Array(w373, w372) -> (w371:refnum<queue>[])
        n173 = Generate User Event(user event=w374, event data cluster=w376) -> ()  [unwired: 2 in, 2 out]
        n174 = for {
          tunnel: w371 -> [w384] mode=indexing
          tunnel: w376 -> [w383]
          n175 = call "Queue In.vi"("First"=TRUE, "Message"=w383, "Queue In"=w384) -> ()  [unwired: 7 in, 2 out]
        }
        n176 = call "Queue Clear.vi"("error in (no error)"=w378, "Queue In"=w380) -> ("error out"=w377:errorcluster, "Queue Out"=w379:refnum<queue>)  [unwired: 8 in]
      }
      frame "Quit" {
      }
    }
    n177 = call "Queue In.vi"("error in (no error)"=w303, "Data"=w301, "Message"=w302, "Queue In"=w306) -> ("error out"=w304:errorcluster, "Queue Out"=w305:refnum<queue>)  [unwired: 6 in]
  }
  n178 = call "000 Driver Message.vi"("Queue In"=w5) -> ("error out"=w24:errorcluster)  [unwired: 8 in, 2 out]
  n179 = call "Queue Release.vi"("error in (no error)"=w21, "Queue In"=w20) -> ("error out"=w23:errorcluster)  [unwired: 9 in]
  n180 = call "Queue Release.vi"("error in (no error)"=w13, "Queue In"=w12) -> ("error out"=w16:errorcluster)  [unwired: 9 in]
  n181 = Unregister For Events(event registration refnum=w10) -> (error out=w11:errorcluster)  [unwired: 1 in]
  n182 = Destroy User Event(user event=w6, error in=w11) -> (error out=w15:errorcluster)
  n183 = Call Chain() -> (call chain=w18:string[])
  n184 = Merge Errors(w15, w16, w24, w23) -> (w17:errorcluster)
  n185 = Array Size(array=w18) -> (size(s)=w19:i32)
  n186 = case shown="2.." w19 {
    tunnel: w17 -> [_ w389]
    frame 0, Default {
    }
    frame 2.. {
      n187 = invoke class="VI" method="FP.Close"(error in=w389) -> ()  [unwired: 2 in, 3 out]
    }
  }
